vi "altitude.vi"(4 "center":cluster{"x":i32, "y":i32}={"x"=35, "y"=32}, 6 "size":i16=29, 7 "altitude":dbl(slide)=9.183673469387756 scale=0.0..100.0, 10 "pict in":picture) -> (3 "pict out":picture)   [LabVIEW 2017]
panel:
  in  "change":dbl
  in  "Old altitude":dbl
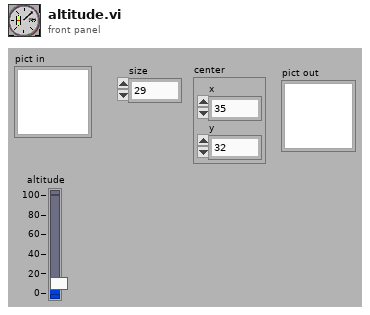
[diagram p1: front panel]
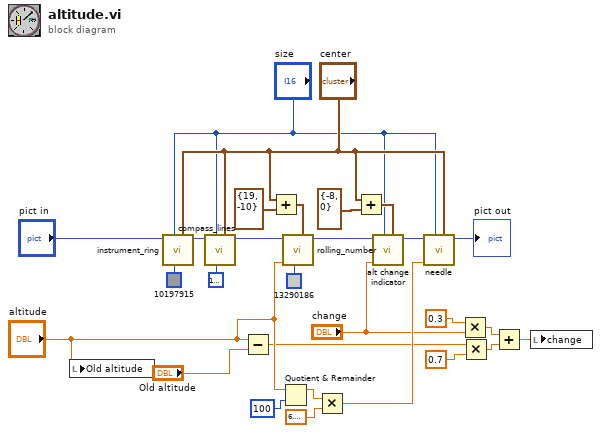
[diagram p0: block diagram]
diagram:
  n1 = local write "Old altitude"("altitude") -> ()
  n2 = call "instrument_ring.vi"("center"="center", "inside color"=u32 10197915, "size"="size", "pict in"="pict in") -> ("new picture"=w24:picture)  [unwired: 6 in]
  n3 = call "compass_lines.vi"("center"="center", "color"=u32 16777222, "size"="size", "pict in"=w24) -> ("pict out"=w23:picture)  [unwired: 6 in]
  n4 = Subtract(x="altitude", y="Old altitude") -> (x-y=w3:dbl)
  n5 = Add(x="center", y=cluster{"x":i32, "y":i32} {"x"=19, "y"=-10} ("center 2")) -> (x+y=w14:cluster{"x":i32, "y":i32})
  n6 = Quotient & Remainder(x="altitude", y=100) -> (x-y*floor(x/y)=w21:dbl)  [unwired: 1 out]
  n7 = call "rolling_number.vi"("Position"=w14, "Background color"=u32 13290186, "number"="altitude", "pict in"=w23) -> ("pict out"=w16:picture)  [unwired: 6 in]
  n8 = Multiply(x=w21, y=6.283185307179586) -> (x*y=w17:dbl)
  n9 = Add(x="center", y=cluster{"x":i32, "y":i32} {"x"=-8, "y"=0} ("center 2")) -> (x+y=w13:cluster{"x":i32, "y":i32})
  n10 = call "alt change indicator.vi"("Cluster"=w13, "size"="size", "change"="change", "pict in"=w16) -> ("pict out"=w19:picture)  [unwired: 6 in]
  n11 = call "needle.vi"("center"="center", "size"="size", "angle"=w17, "pict in"=w19) -> ("pict out"=→"pict out":picture)  [unwired: 6 in]
  n12 = Multiply(x=0.3, y="change") -> (x*y=w6:dbl)
  n13 = Multiply(x=w3, y=0.7) -> (x*y=w2:dbl)
  n14 = Add(x=w6, y=w2) -> (x+y=w1:dbl)
  n15 = local write "change"(w1) -> ()
